vi "Camera_SetCameraRing.vi"(8 "error in (no error)":errorcluster, 10 "Camera Index":u16, 11 "CameraName":refnum<vi>) -> (0 "error out":errorcluster)   [LabVIEW 2019]
uses:
  <vilib>/userdefined/High Color/IMAQdx.ctl
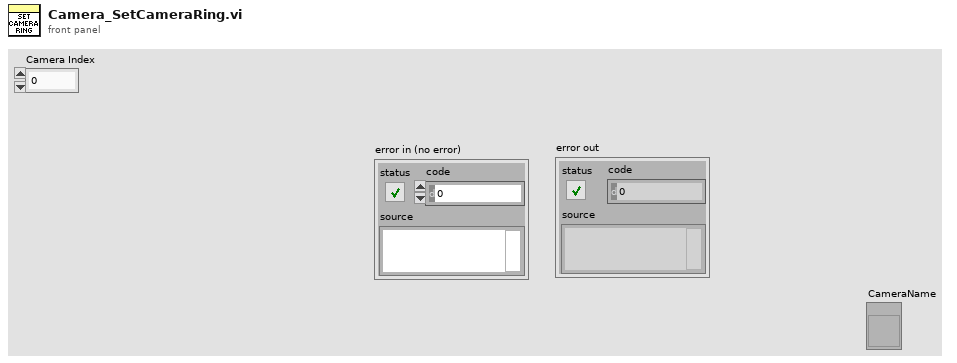
[diagram p1: front panel]
types:
  T1 = enum16{"Init", "Grab", "Get All", "Close", "Set Camera"}
  T2 = typedef "IMAQdx.ctl" = refnum<k21>
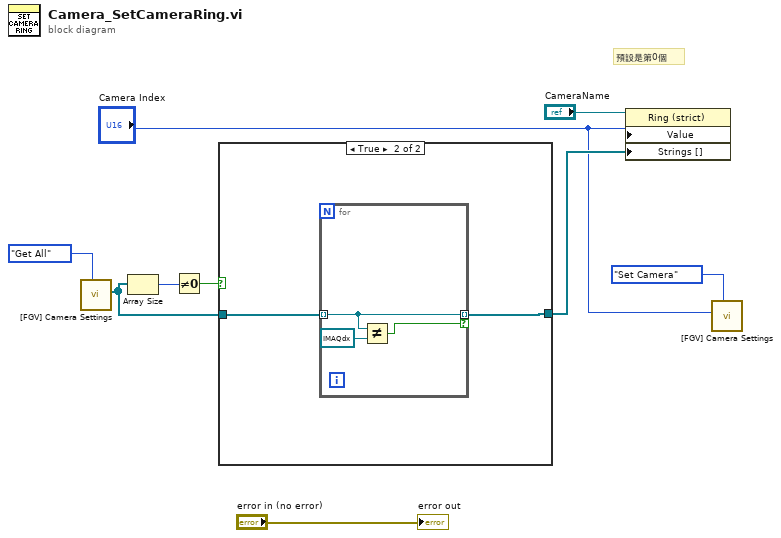
[diagram p0: block diagram]
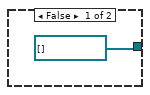
[diagram p2: hidden frame]
diagram:
  # "預設是第0個"
  n1 = call "[FGV] Camera Settings.vi"("Action"=T1."Get All") -> ("Camera Interface Name"=w3:T2[])  [unwired: 8 in, 2 out]
  n2 = Array Size(array=w3) -> (size(s)=w9:i32)
  n3 = Not Equal To 0?(x=w9) -> (x != 0?=w8:bool)
  n4 = case shown="True" w8 {
    tunnel: w3 -> [_ w11]
    tunnel: [T2[] [] w12] -> w6
    frame False {
    }
    frame True {
      n5 = for {
        tunnel: [w15] -> w12 mode=indexing if=w13
        tunnel: w11 -> [w15] mode=indexing
        n6 = Not Equal?(x=w15, y=T2 refnum) -> (x != y?=w13:bool)
      }
    }
  }
  n7 = property class="Ring (strict)"(reference="CameraName", "Value"="Camera Index", "Strings []"=w6) -> ()  [unwired: 1 in, 2 out]
  n8 = call "[FGV] Camera Settings.vi"("Action"=T1."Set Camera", "Value"="Camera Index") -> ()  [unwired: 7 in, 3 out]
  "error out" <- "error in (no error)"
